vi "InitializeAnalogOutputforPAD.vi"(0 "AOTF":u16(ring) items=["None", "Laser 1", "Laser 2", "Laser 1 + 2", "Laser 3", "Laser 1 + 3", "Laser 2 + 3", "Laser 1+2+3", "Laser 1+2+3+4", "Laser 2+3+4"], 1 "% puls-duration":dbl=95.0, 2 "% rel. duration":u8=50 min=1 max=99, 3 "EOM":u16(ring) items=["None", "Trace", "Retrace", "All"]) -> ()   [LabVIEW 2009]
uses:
  ImageSettings.ctt
  TimingInfo.ctt
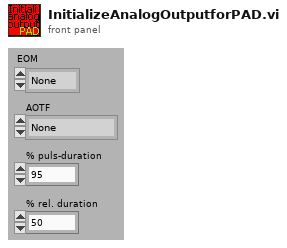
[diagram p1: front panel]
types:
  T1 = typedef "ImageSettings.ctt" = cluster{"Start Position (µm)":cluster{"x":dbl, "y":dbl, "z":dbl}, "End Position (µm)":cluster{"x":dbl, "y":dbl, "z":dbl}, "Image Resolution (nm/pixel)":cluster{"x":dbl, "y":dbl, "z":dbl}, "Image Size (µm)":cluster{"x":dbl, "y":dbl, "z":dbl}, "Image Size (pixel)":cluster{"x":u32, "y":u32, "z":u32}, "Time Resolution\n(ms/pixel)":dbl, "1st Axis":u16, "2nd Axis":u16, "Retrace":bool, "Estimated Time":string}
  T2 = typedef "TimingInfo.ctt" = cluster{"Fs":dbl, "#s":dbl}
  T3 = typedef "EOMSettings.ctt" = cluster{"Output Channel":tag, "EOM Voltage":dbl, "Pixel per Polymode Cycle":u32, "Time per Polymode Cycle":dbl}
  T4 = typedef "AnalogSettings.ctt" = cluster{"PCI 671x Device Number":u32, "Samples per Unit":u32}
  T5 = typedef "AOTFSettings.ctt" = cluster{"Laser 1 Output Channel":tag, "AOTF  1 Output Voltage":dbl, "Laser 2 Output Channel":tag, "AOTF  2 Output Voltage":dbl, "Laser 3 Output Channel":tag, "AOTF  3 Output Voltage":dbl, "Pixel per Cycle":u16, "Time per Cycle  / ms":dbl, "Laser 4 Output Channel":tag, "AOTF  4 Output Voltage":dbl}
  T6 = typedef "AnalogTrace.ctt" = cluster{"Used":bool, "Waveform":waveform(dbl)}
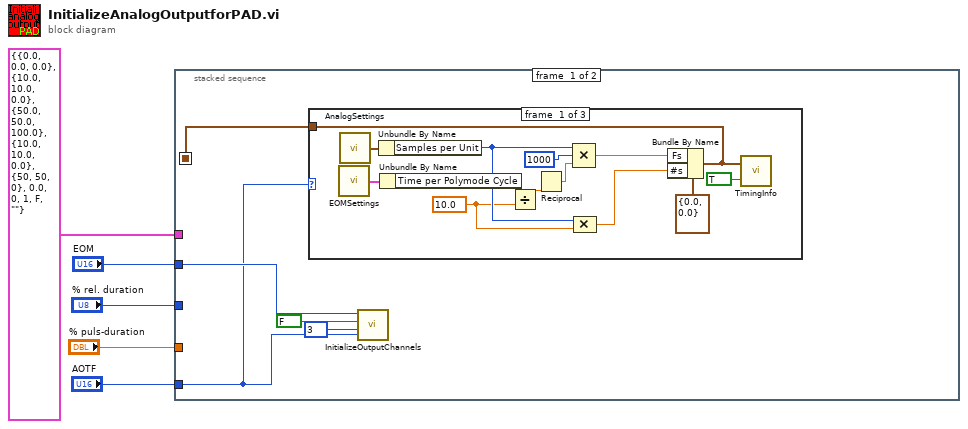
[diagram p0: block diagram]
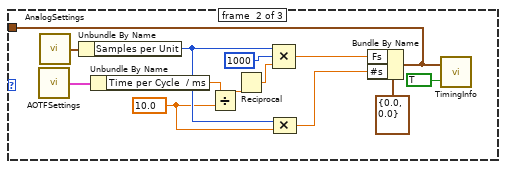
[diagram p2: hidden frame]
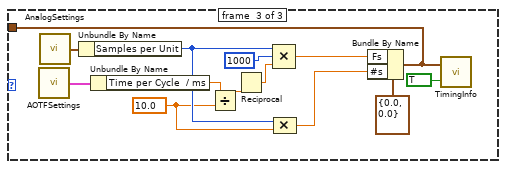
[diagram p3: hidden frame]
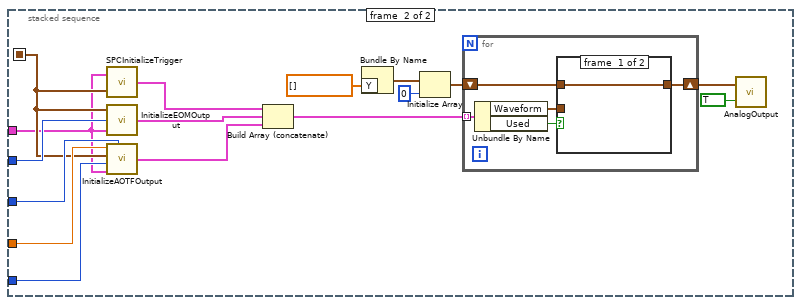
[diagram p4: hidden frame]
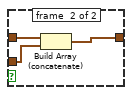
[diagram p5: hidden frame]
diagram:
  n1 = stacked-sequence {
    seq-local: [w8 _] -> [_ w51]
    tunnel: T1 {"Start Position (µm)"={"x"=0.0, "y"=0.0, "z"=0.0}, "End Position (µm)"={"x"=10.0, "y"=10.0, "z"=0.0}, "Image Resolution (nm/pixel)"={"x"=50.0, "y"=50.0, "z"=100.0}, "Image Size (µm)"={"x"=10.0, "y"=10.0, "z"=0.0}, "Image Size (pixel)"={"x"=50, "y"=50, "z"=0}, "Time Resolution\n(ms/pixel)"=0.0, "1st Axis"=0, "2nd Axis"=1, "Retrace"=FALSE, "Estimated Time"=""} ("Image Settings") -> [_ w50]
    tunnel: "EOM" -> [w7 w59]
    tunnel: "AOTF" -> [w6 w56]
    tunnel: "% puls-duration" -> [_ w53]
    tunnel: "% rel. duration" -> [_ w52]
    frame #0 {
      w9 = u16 3 items=["x", "y", "z", ""] ("1st Axis")
      n2 = case shown="7" w6 {
        tunnel: [w11 w25 w38] -> w8
        frame #0 {
          w12 = 10.0 ("y")
          n3 = call "EOMSettings.vi"() -> ("EOM Settings (output)"=w23:T3)  [unwired: 2 in]
          n4 = call "AnalogSettings.vi"() -> ("Analog Settings (output)"=w20:T4)  [unwired: 2 in]
          n5 = Unbundle By Name(w20) -> ("Samples per Unit"=w16:u32)
          n6 = Unbundle By Name(w23) -> ("Time per Polymode Cycle"=w13:dbl)
          n7 = Divide(x=w13, y=w12) -> (x/y=w14:dbl)
          n8 = Reciprocal(x=w14) -> (1/x=w17:dbl)
          n9 = Compound Arithmetic op=MULTIPLY(w16, u32 1000 ("value"), w17) -> (w18:dbl)
          n10 = Compound Arithmetic op=MULTIPLY(w16, w12) -> (w15:dbl)
          n11 = Bundle By Name(cluster=T2 {"Fs"=0.0, "#s"=0.0} ("Timing Info"), "Fs"=w18, "#s"=w15) -> (w11:T2)
          n12 = call "TimingInfo.vi"("Get/Set"=TRUE, "Timing Info (input)"=w11) -> ()  [unwired: 1 out]
        }
        frame #1 {
          w26 = 10.0 ("y")
          n13 = call "AOTFSettings.vi"() -> ("AOTF Setting (Output)"=w24:T5)  [unwired: 2 in]
          n14 = call "AnalogSettings.vi"() -> ("Analog Settings (output)"=w34:T4)  [unwired: 2 in]
          n15 = Unbundle By Name(w34) -> ("Samples per Unit"=w30:u32)
          n16 = Unbundle By Name(w24) -> ("Time per Cycle  / ms"=w27:dbl)
          n17 = Divide(x=w27, y=w26) -> (x/y=w28:dbl)
          n18 = Reciprocal(x=w28) -> (1/x=w31:dbl)
          n19 = Compound Arithmetic op=MULTIPLY(w30, u32 1000 ("value"), w31) -> (w32:dbl)
          n20 = Compound Arithmetic op=MULTIPLY(w30, w26) -> (w29:dbl)
          n21 = Bundle By Name(cluster=T2 {"Fs"=0.0, "#s"=0.0} ("Timing Info"), "Fs"=w32, "#s"=w29) -> (w25:T2)
          n22 = call "TimingInfo.vi"("Get/Set"=TRUE, "Timing Info (input)"=w25) -> ()  [unwired: 1 out]
        }
        frame #2 {
          w39 = 10.0 ("y")
          n23 = call "AOTFSettings.vi"() -> ("AOTF Setting (Output)"=w37:T5)  [unwired: 2 in]
          n24 = call "AnalogSettings.vi"() -> ("Analog Settings (output)"=w47:T4)  [unwired: 2 in]
          n25 = Unbundle By Name(w47) -> ("Samples per Unit"=w43:u32)
          n26 = Unbundle By Name(w37) -> ("Time per Cycle  / ms"=w40:dbl)
          n27 = Divide(x=w40, y=w39) -> (x/y=w41:dbl)
          n28 = Reciprocal(x=w41) -> (1/x=w44:dbl)
          n29 = Compound Arithmetic op=MULTIPLY(w43, u32 1000 ("value"), w44) -> (w45:dbl)
          n30 = Compound Arithmetic op=MULTIPLY(w43, w39) -> (w42:dbl)
          n31 = Bundle By Name(cluster=T2 {"Fs"=0.0, "#s"=0.0} ("Timing Info"), "Fs"=w45, "#s"=w42) -> (w38:T2)
          n32 = call "TimingInfo.vi"("Get/Set"=TRUE, "Timing Info (input)"=w38) -> ()  [unwired: 1 out]
        }
      }
      n33 = call "InitializeOutputChannels.vi"("AOTF"=w6, "1st Axis"=w9, "Retrace"=FALSE, "EOM"=w7) -> ()
    }
    frame #1 {
      n34 = call "SPCInitializeTrigger.vi"("timing info"=w51, "Image Settings"=w50) -> ("signal out"=w58:T6)
      n35 = call "InitializeEOMOutput.vi"("Image Settings"=w50, "EOM"=w59, "Timing Info"=w51) -> ("Analog Output"=w54:T6)
      n36 = call "InitializeAOTFOutput.vi"("% puls-duration"=w53, "Timing Info"=w51, "AOTF"=w56, "Image Settings"=w50, "% rel. duration"=w52) -> ("Array"=w55:T6[])
      n37 = Build Array (concatenate)(w58, w54, w55) -> (w64:T6[])
      n38 = Bundle By Name("Y"=dbl[] []) -> (w61:waveform(dbl))  [unwired: 1 in]
      n39 = Initialize Array(w61, 0 ("dimension size")) -> (w60:waveform(dbl)[])
      n40 = for {
        shift-right: [w68] -> w57
        shift-left: w60 -> [w67]
        tunnel: w64 -> [w70] mode=indexing
        n41 = Unbundle By Name(w70) -> ("Waveform"=w66:waveform(dbl), "Used"=w69:bool)
        n42 = case shown="False" w69 {
          tunnel: [w71 w74] -> w68
          tunnel: w67 -> [w71 w73]
          tunnel: w66 -> [_ w72]
          frame #0 {
          }
          frame #1 {
            n43 = Build Array (concatenate)(w73, w72) -> (w74:waveform(dbl)[])
          }
        }
      }
      n44 = call "AnalogOutput.vi"("Get/Set"=TRUE, "Analog Output (input)"=w57) -> ()  [unwired: 1 out]
    }
  }
